vi "Begin.vi"(8 "error in (no error)":errorcluster, 10 "Settings":variant, 11 "Elevator Concrete in":refnum<class "Elevator Arm.lvclass">) -> (0 "error out":errorcluster, 3 "Elevator Concrete out":refnum<class "Elevator Arm.lvclass">)   [LabVIEW 2018, in "Elevator.lvlib" / "Elevator Arm.lvclass"]
doc: "Opens references and configures Elevator Arm resources."
uses:
  Elevator Arm.lvclass
  C:/Users/Public/Documents/2019DeepSpace/Classes/Elevator/Elevator.lvclass
  <vilib>/Rock Robotics/WPI/ThirdParty/Phoenix-LabVIEW/Motor Controller/Controls/CTRE_Phoenix_MotorControl_EnhancedMotorControllerConfigurables.ctl
  <vilib>/Rock Robotics/WPI/ThirdParty/Phoenix-LabVIEW/Motor Controller/Controls/CTRE_Phoenix_MotorControl_BaseConfigurables.ctl
  <vilib>/Rock Robotics/WPI/ThirdParty/Phoenix-LabVIEW/Motor Controller/Controls/CTRE_Phoenix_MotorControl_VelocityMeasurementPeriod.ctl
  <vilib>/Rock Robotics/WPI/ThirdParty/Phoenix-LabVIEW/Motor Controller/Controls/CTRE_Phoenix_MotorControl_SlotStructure.ctl
  <vilib>/Rock Robotics/WPI/ThirdParty/Phoenix-LabVIEW/Motor Controller/Controls/CTRE_Phoenix_MotorControl_FilterStruct.ctl
  <vilib>/Rock Robotics/WPI/ThirdParty/Phoenix-LabVIEW/Motor Controller/Controls/CTRE_Phoenix_MotorControl_RemoteSourceType.ctl
  <vilib>/Rock Robotics/WPI/ThirdParty/Phoenix-LabVIEW/Controls/CTRE_Phoenix_CustomParamConfiguration.ctl
  <vilib>/Rock Robotics/WPI/ThirdParty/Phoenix-LabVIEW/Motor Controller/Controls/CTRE_Phoenix_MotorControl_FeedbackDevice.ctl
  <vilib>/Rock Robotics/WPI/ThirdParty/Phoenix-LabVIEW/Motor Controller/Controls/CTRE_Phoenix_MotorControl_SensorTermFeedbackDevice_Enhanced.ctl
  <vilib>/Rock Robotics/WPI/ThirdParty/Phoenix-LabVIEW/Motor Controller/Controls/CTRE_Phoenix_MotorControl_LimitSwitchNormal.ctl
  <vilib>/Rock Robotics/WPI/ThirdParty/Phoenix-LabVIEW/Motor Controller/Controls/CTRE_Phoenix_MotorControl_LimitSwitchSource_Local.ctl
  Controls/Elevator Position.ctl
  Elevator Arm.lvclass/Elevator Arm.ctl
  Elevator.lvclass/Elevator.ctl
  Public Methods/Write Array.vi
  <vilib>/Rock Robotics/WPI/ThirdParty/Phoenix-LabVIEW/Motor Controller/Get/CTRE_Phoenix_MotorController_GetPulseWidthAll.vi
  Elevator.lvclass
panel:
  out "Pulse Width Rise-to-Rise Time (us)":i32
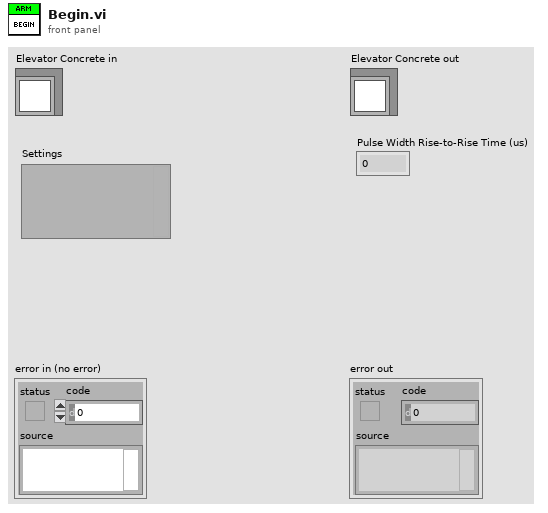
[diagram p1: front panel]
types:
  T1 = typedef "Elevator.lvlib/Elevator.lvclass/Elevator Position.ctl" = enum16{"CS, Cargo Ship Cargo", "C0, Cargo Ground", "C1, LV1 Cargo", "C2, LV2 Cargo", "C3, LV3 Cargo", "H0, LV1 Hatch", "H1, LV2 Hatch", "H2, LV3 Hatch"}
  T2 = typedef "CTRE_Phoenix_MotorControl_EnhancedMotorControllerConfigurables.ctl" = cluster{"Base Configurables":T3, "primaryPID":cluster{"selectedFeedbackCoefficient":dbl, "selectedFeedbackSensor":T9}, "auxiliaryPID":cluster{"selectedFeedbackCoefficient":dbl, "selectedFeedbackSensor":T9}, "sum0Term":T10, "sum1Term":T10, "diff0Term":T10, "diff1Term":T10, "forwardLimitSwitchNormal":T11, "reverseLimitSwitchNormal":T11, "forwardLimitSwitchDeviceID":i32, "reverseLimitSwitchDeviceID":i32, "forwardLimitSwitchSource":T12, "reverseLimitSwitchSource":T12, "peakCurrentLimit":i32, "peakCurrentDuration":i32, "continuousCurrentLimit":i32}
  T3 = typedef "CTRE_Phoenix_MotorControl_BaseConfigurables.ctl" = cluster{"openLoopRamp":dbl, "closedLoopRamp":dbl, "peakOutputForward":dbl, "peakOutputReverse":dbl, "nominalOutputForward":dbl, "nominalOutputReverse":dbl, "neutralDeadband":dbl, "voltageCompSaturation":dbl, "voltageMeasurementFilter":i32, "velocityMeasurementPeriod":T4, "velocityMeasurementWindow":i32, "forwardSoftLimitThreshold":i32, "reverseSoftLimitThreshold":i32, "forwardSoftLimitEnable":bool, "reverseSoftLimitEnable":bool, "slot0":T5, "slot1":T5, "slot2":T5, "slot3":T5, "auxPIDPolarity":bool, "remoteFilter0":T6, "remoteFilter1":T6, "motionCruiseVelocity":i32, "motionAcceleration":i32, "motionProfileTrajectoryPeriod":i32, "feedbackNotContinuous":bool, "remoteSensorClosedLoopDisableNeutralOnLOS":bool, "clearPositionOnLimitF":bool, "clearPositionOnLimitR":bool, "clearPositionOnQuadIdx":bool, "limitSwitchDisableNeutralOnLOS":bool, "softLimitDisableNeutralOnLOS":bool, "pulseWidthPeriod_EdgesPerRot":i32, "pulseWidthPeriod_FilterWindowSz":i32, "customParam":T8, "trajectoryInterpolationEnable":bool}
  T4 = typedef "CTRE_Phoenix_MotorControl_VelocityMeasurementPeriod.ctl" = u16
  T5 = typedef "CTRE_Phoenix_MotorControl_SlotStructure.ctl" = cluster{"P":dbl, "I":dbl, "D":dbl, "F":dbl, "integralZone":dbl, "allowableClosedLoopError":i32, "maxIntegralAccumulator":dbl, "closedLoopPeakOutput":dbl, "closedLoopPeriod":i32}
  T6 = typedef "CTRE_Phoenix_MotorControl_FilterStruct.ctl" = cluster{"remoteSensorDeviceID":u8, "remoteSensorSource":T7}
  T7 = typedef "CTRE_Phoenix_MotorControl_RemoteSourceType.ctl" = enum16{"Off", "Talon SRX Selected Sensor", "Pigeon IMU Yaw", "Pigeon IMU Pitch", "Pigeon IMU Roll", "CANifier Quadrature", "CANifier PWM Input 0", "CANifier PWM Input 1", "CANifier PWM Input 2", "CANifier PWM Input 3", "Gadgeteer Pigeon Yaw", "Gadgeteer Pigeon Pitch", "Gadgeteer Pigeon Roll"}
  T8 = typedef "CTRE_Phoenix_CustomParamConfiguration.ctl" = cluster{"customParam0":i32, "customParam1":i32}
  T9 = typedef "CTRE_Phoenix_MotorControl_FeedbackDevice.ctl" = i8
  T10 = typedef "CTRE_Phoenix_MotorControl_SensorTermFeedbackDevice_Enhanced.ctl" = i8
  T11 = typedef "CTRE_Phoenix_MotorControl_LimitSwitchNormal.ctl" = enum16{"Normally Open", "Normally Closed", "Disabled"}
  T12 = typedef "CTRE_Phoenix_MotorControl_LimitSwitchSource_Local.ctl" = enum16{"Feedback Connector", "Remote Talon SRX", "Remote CANifier", "Deactivated"}
  T13 = typedef "Elevator.lvlib/Elevator.lvclass/Elevator IDs.ctl" = cluster{"Wrist":u8, "Left Master":u8, "Left Slave":u8, "Right Master":u8, "Right Slave":u8, "Vacumm Pump 1":u8, "Vacumm Pump 2":u8, "Elevator Linear Master":u8, "Elevator Linear Slave":u8}
  T14 = typedef "Elevator.lvlib/Elevator.lvclass/Elevator Constants.ctl" = cluster{"Arm Motion Magic Max Velocity":u32, "Arm Motion Magic Max Acceleration":u32, "Wrist Motion Magic Max Velocity":u32, "Wrist Motion Magic Max Acceleration":u32, "Elevator Linear Motion Magic Max Velocity":u32, "Elevator Linear Motion Magic Max Acceleration":u32, "Arm Gear Ratio":dbl, "Wrist Gear Ratio":dbl, "Elevator Linear Gear Ratio":dbl, "Arm Encoder ABS Value":i32, "Wrist Encoder ABS Value":i32}
  T15 = typedef "WPI_MotorControlDeviceRef.ctl" = cluster{"DeviceStatus":errorcluster, "Type":T16, "PWM":cluster{"PWM Channel":T17, "DeadBand":T18}, "CAN":cluster{"Device Number":u8, "SetOutput VI Ref":variant, "GetOutput VI Ref":variant, "Enable VI Ref":variant, "Disable VI Ref":variant, "Data":variant}, "Invert":bool, "DIO PWM":cluster{"PWM \"Enable\" Channel":T17, "DIOChannel":T19, "PWM Rate":dbl}}
  T16 = typedef "WPI_MotorControlType.ctl" = enum16{"PWM", "CAN", "DIO PWM"}
  T17 = typedef "FPGA_DIOPWMChannel.ctl" = enum8{"PWM 0", "PWM 1", "PWM 2", "PWM 3", "PWM 4", "PWM 5", "PWM 6", "PWM 7", "PWM 8", "PWM 9", "PWM MXP 0", "PWM MXP 1", "PWM MXP 2", "PWM MXP 3", "PWM MXP 4", "PWM MXP 5", "PWM MXP 6", "PWM MXP 7", "PWM MXP 8", "PWM MXP 9", "Invalid"}
  T18 = typedef "WPI_PWMDeadband.ctl" = cluster{"Name":string, "maxPositivePwm":i32, "minPositivePwm":i32, "centerPwm":i32, "maxNegativePwm":i32, "minNegativePwm":i32, "angularRange":u16}
  T19 = typedef "FPGA_DIOChannel.ctl" = enum8{"DIO 0", "DIO 1", "DIO 2", "DIO 3", "DIO 4", "DIO 5", "DIO 6", "DIO 7", "DIO 8", "DIO 9", "DIO MXP 0", "DIO MXP 1", "DIO MXP 2", "DIO MXP 3", "DIO MXP 4", "DIO MXP 5", "DIO MXP 6", "DIO MXP 7", "DIO MXP 8", "DIO MXP 9", "DIO MXP 10", "DIO MXP 11", "DIO MXP 12", "DIO MXP 13", "DIO MXP 14", "DIO MXP 15", "SPI Port CS1", "SPI Port CS2", "SPI Port CS3", "SPI Port MISO", "SPI Port MOSI", "Invalid"}
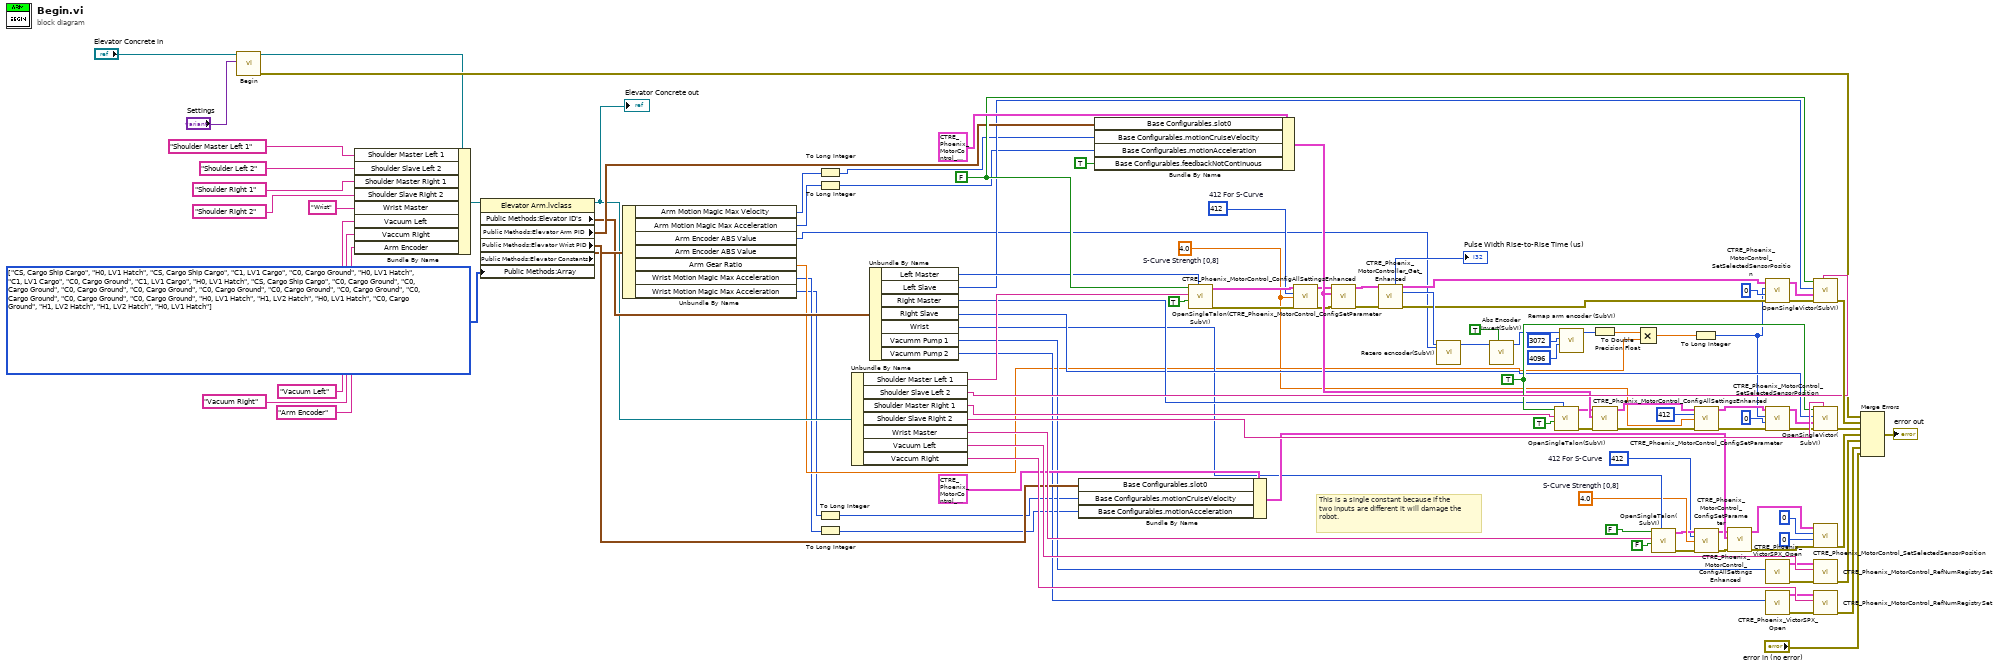
[diagram p0: block diagram]
diagram:
  w12 = T1[][] [[enum."CS, Cargo Ship Cargo", enum."H0, LV1 Hatch", enum."CS, Cargo Ship Cargo", enum."C1, LV1 Cargo"], [enum."C0, Cargo Ground", enum."H0, LV1 Hatch", enum."C1, LV1 Cargo", enum."C0, Cargo Ground"], [enum."C1, LV1 Cargo", enum."H0, LV1 Hatch", enum."CS, Cargo Ship Cargo", enum."C0, Cargo Ground"], [enum."C0, Cargo Ground", enum."C0, Cargo Ground", enum."C0, Cargo Ground", enum."C0, Cargo Ground"], [enum."C0, Cargo Ground", enum."C0, Cargo Ground", enum."C0, Cargo Ground", enum."C0, Cargo Ground"], [enum."C0, Cargo Ground", enum."H0, LV1 Hatch", enum."H1, LV2 Hatch", enum."H0, LV1 Hatch"], [enum."C0, Cargo Ground", enum."H1, LV2 Hatch", enum."H1, LV2 Hatch", enum."H0, LV1 Hatch"]] items=["CS, Cargo Ship Cargo", "C0, Cargo Ground", "C1, LV1 Cargo", "C2, LV2 Cargo", "C3, LV3 Cargo", "H0, LV1 Hatch", "H1, LV2 Hatch", "H2, LV3 Hatch"] ("Array")
  w22 = u16 412  # 412 For S-Curve
  w23 = u32 412  # 412 For S-Curve
  w31 = 4.0  # S-Curve Strength [0,8]
  w1 = 4.0  # S-Curve Strength [0,8]
  w72 = FALSE ("invert")
  w88 = TRUE ("Invert?")
  # "This is a single constant because if the two inputs are different it will damage the robot."
  n1 = call-parent "Begin.vi"("Settings"="Settings", "Elevator in"="Elevator Concrete in") -> ("error out"=w16:errorcluster, "Elevator out"=w14:refnum<class "Elevator Arm.lvclass">)  [unwired: 8 in]
  n2 = Bundle By Name(cluster=w14, "Shoulder Master Left 1"="Shoulder Master Left 1" ("Shoulder Slave Left 1"), "Shoulder Slave Left 2"="Shoulder Left 2", "Shoulder Master Right 1"="Shoulder Right 1", "Shoulder Slave Right 2"="Shoulder Right 2", "Wrist Master"="Wrist", "Vacuum Left"="Vacuum Left", "Vaccum Right"="Vacuum Right", "Arm Encoder"="Arm Encoder") -> (w67:refnum<class "Elevator Arm.lvclass">)
  n3 = property class="Elevator Arm.lvclass"(reference=w67, "Public Methods:Array"=w12) -> (reference out=w13:refnum<class "Elevator Arm.lvclass">, "Public Methods:Elevator ID's"=w61:T13, "Public Methods:Elevator Arm PID"=w66:T5, "Public Methods:Elevator Wrist PID"=w65:T5, "Public Methods:Elevator Constants"=w64:T14)  [unwired: 1 in, 1 out]
  "Elevator Concrete out" <- w13
  n4 = Unbundle By Name(w64) -> ("Arm Motion Magic Max Velocity"=w63:u32, "Arm Motion Magic Max Acceleration"=w62:u32, "Arm Encoder ABS Value"=w4:i32, "Arm Gear Ratio"=w5:dbl, "Wrist Motion Magic Max Acceleration"=w3:u32, "Wrist Motion Magic Max Acceleration"=w2:u32)  [unwired: 1 out]
  n5 = To Long Integer(number=w63) -> (32bit integer=w9:i32)
  n6 = To Long Integer(number=w62) -> (32bit integer=w8:i32)
  n7 = To Long Integer(number=w2) -> (32bit integer=w6:i32)
  n8 = To Long Integer(number=w3) -> (32bit integer=w7:i32)
  n9 = Unbundle By Name(w13) -> ("Shoulder Master Left 1"=w106:string, "Shoulder Slave Left 2"=w105:string, "Shoulder Master Right 1"=w104:string, "Shoulder Slave Right 2"=w103:string, "Wrist Master"=w102:string, "Vacuum Left"=w101:string, "Vaccum Right"=w100:string)
  n10 = Unbundle By Name(w61) -> ("Left Master"=w58:u8, "Left Slave"=w57:u8, "Right Master"=w56:u8, "Right Slave"=w55:u8, "Wrist"=w54:u8, "Vacumm Pump 1"=w59:u8, "Vacumm Pump 2"=w60:u8)
  n11 = Bundle By Name(cluster=T2 {"Base Configurables"={"openLoopRamp"=0.0, "closedLoopRamp"=0.0, "peakOutputForward"=1.0, "peakOutputReverse"=-1.0, "nominalOutputForward"=0.0, "nominalOutputReverse"=0.0, "neutralDeadband"=0.04, "voltageCompSaturation"=0.0, "voltageMeasurementFilter"=32, "velocityMeasurementPeriod"=100, "velocityMeasurementWindow"=64, "forwardSoftLimitThreshold"=0, "reverseSoftLimitThreshold"=0, "forwardSoftLimitEnable"=FALSE, "reverseSoftLimitEnable"=FALSE, "slot0"={"P"=0.0, "I"=0.0, "D"=0.0, "F"=0.0, "integralZone"=0.0, "allowableClosedLoopError"=0, "maxIntegralAccumulator"=0.0, "closedLoopPeakOutput"=1.0, "closedLoopPeriod"=1}, "slot1"={"P"=0.0, "I"=0.0, "D"=0.0, "F"=0.0, "integralZone"=0.0, "allowableClosedLoopError"=0, "maxIntegralAccumulator"=0.0, "closedLoopPeakOutput"=1.0, "closedLoopPeriod"=1}, "slot2"={"P"=0.0, "I"=0.0, "D"=0.0, "F"=0.0, "integralZone"=0.0, "allowableClosedLoopError"=0, "maxIntegralAccumulator"=0.0, "closedLoopPeakOutput"=1.0, "closedLoopPeriod"=1}, "slot3"={"P"=0.0, "I"=0.0, "D"=0.0, "F"=0.0, "integralZone"=0.0, "allowableClosedLoopError"=0, "maxIntegralAccumulator"=0.0, "closedLoopPeakOutput"=1.0, "closedLoopPeriod"=1}, "auxPIDPolarity"=FALSE, "remoteFilter0"={"remoteSensorDeviceID"=0, "remoteSensorSource"=enum."Off"}, "remoteFilter1"={"remoteSensorDeviceID"=0, "remoteSensorSource"=enum."Off"}, "motionCruiseVelocity"=0, "motionAcceleration"=0, "motionProfileTrajectoryPeriod"=0, "feedbackNotContinuous"=FALSE, "remoteSensorClosedLoopDisableNeutralOnLOS"=FALSE, "clearPositionOnLimitF"=FALSE, "clearPositionOnLimitR"=FALSE, "clearPositionOnQuadIdx"=FALSE, "limitSwitchDisableNeutralOnLOS"=FALSE, "softLimitDisableNeutralOnLOS"=FALSE, "pulseWidthPeriod_EdgesPerRot"=1, "pulseWidthPeriod_FilterWindowSz"=1, "customParam"={"customParam0"=0, "customParam1"=0}, "trajectoryInterpolationEnable"=TRUE}, "primaryPID"={"selectedFeedbackCoefficient"=1.0, "selectedFeedbackSensor"=0}, "auxiliaryPID"={"selectedFeedbackCoefficient"=1.0, "selectedFeedbackSensor"=0}, "sum0Term"=0, "sum1Term"=0, "diff0Term"=0, "diff1Term"=0, "forwardLimitSwitchNormal"=enum."Normally Open", "reverseLimitSwitchNormal"=enum."Normally Open", "forwardLimitSwitchDeviceID"=0, "reverseLimitSwitchDeviceID"=0, "forwardLimitSwitchSource"=enum."Feedback Connector", "reverseLimitSwitchSource"=enum."Feedback Connector", "peakCurrentLimit"=1, "peakCurrentDuration"=1, "continuousCurrentLimit"=1} ("Enhanced Motor Controller Configurables"), "Base Configurables.slot0"=w65, "Base Configurables.motionCruiseVelocity"=w6, "Base Configurables.motionAcceleration"=w7) -> (w75:T2)
  n12 = Bundle By Name(cluster=T2 {"Base Configurables"={"openLoopRamp"=0.0, "closedLoopRamp"=0.0, "peakOutputForward"=1.0, "peakOutputReverse"=-1.0, "nominalOutputForward"=0.0, "nominalOutputReverse"=0.0, "neutralDeadband"=0.04, "voltageCompSaturation"=0.0, "voltageMeasurementFilter"=32, "velocityMeasurementPeriod"=100, "velocityMeasurementWindow"=64, "forwardSoftLimitThreshold"=0, "reverseSoftLimitThreshold"=0, "forwardSoftLimitEnable"=FALSE, "reverseSoftLimitEnable"=FALSE, "slot0"={"P"=0.0, "I"=0.0, "D"=0.0, "F"=0.0, "integralZone"=0.0, "allowableClosedLoopError"=0, "maxIntegralAccumulator"=0.0, "closedLoopPeakOutput"=1.0, "closedLoopPeriod"=1}, "slot1"={"P"=0.0, "I"=0.0, "D"=0.0, "F"=0.0, "integralZone"=0.0, "allowableClosedLoopError"=0, "maxIntegralAccumulator"=0.0, "closedLoopPeakOutput"=1.0, "closedLoopPeriod"=1}, "slot2"={"P"=0.0, "I"=0.0, "D"=0.0, "F"=0.0, "integralZone"=0.0, "allowableClosedLoopError"=0, "maxIntegralAccumulator"=0.0, "closedLoopPeakOutput"=1.0, "closedLoopPeriod"=1}, "slot3"={"P"=0.0, "I"=0.0, "D"=0.0, "F"=0.0, "integralZone"=0.0, "allowableClosedLoopError"=0, "maxIntegralAccumulator"=0.0, "closedLoopPeakOutput"=1.0, "closedLoopPeriod"=1}, "auxPIDPolarity"=FALSE, "remoteFilter0"={"remoteSensorDeviceID"=0, "remoteSensorSource"=enum."Off"}, "remoteFilter1"={"remoteSensorDeviceID"=0, "remoteSensorSource"=enum."Off"}, "motionCruiseVelocity"=0, "motionAcceleration"=0, "motionProfileTrajectoryPeriod"=0, "feedbackNotContinuous"=FALSE, "remoteSensorClosedLoopDisableNeutralOnLOS"=FALSE, "clearPositionOnLimitF"=FALSE, "clearPositionOnLimitR"=FALSE, "clearPositionOnQuadIdx"=FALSE, "limitSwitchDisableNeutralOnLOS"=FALSE, "softLimitDisableNeutralOnLOS"=FALSE, "pulseWidthPeriod_EdgesPerRot"=1, "pulseWidthPeriod_FilterWindowSz"=1, "customParam"={"customParam0"=0, "customParam1"=0}, "trajectoryInterpolationEnable"=TRUE}, "primaryPID"={"selectedFeedbackCoefficient"=1.0, "selectedFeedbackSensor"=0}, "auxiliaryPID"={"selectedFeedbackCoefficient"=1.0, "selectedFeedbackSensor"=0}, "sum0Term"=0, "sum1Term"=0, "diff0Term"=0, "diff1Term"=0, "forwardLimitSwitchNormal"=enum."Normally Open", "reverseLimitSwitchNormal"=enum."Normally Open", "forwardLimitSwitchDeviceID"=0, "reverseLimitSwitchDeviceID"=0, "forwardLimitSwitchSource"=enum."Feedback Connector", "reverseLimitSwitchSource"=enum."Feedback Connector", "peakCurrentLimit"=1, "peakCurrentDuration"=1, "continuousCurrentLimit"=1} ("Enhanced Motor Controller Configurables"), "Base Configurables.slot0"=w66, "Base Configurables.motionCruiseVelocity"=w9, "Base Configurables.motionAcceleration"=w8, "Base Configurables.feedbackNotContinuous"=TRUE) -> (w86:T2)
  n13 = call "OpenSingleTalon(SubVI).vi"("can_id"=w58, "sensor_phase"=TRUE, "refnum name"=w106, "invert"=w72) -> ("error out"=w37:errorcluster, "PhoenixMotorControlDevRef"=w39:T15)  [unwired: 6 in]
  n14 = call <vilib>:"CTRE_Phoenix_MotorControl_ConfigSetParameter.vi"("PhoenixMotorControlDevRef"=w39, "Parameter"=w22, "value"=w1, "error in (no error)"=w37) -> ("PhoenixMotorControlDevRef"=w38:T15, "error out"=w36:errorcluster)  [unwired: 10 in]
  n15 = call <vilib>:"CTRE_Phoenix_MotorControl_ConfigAllSettingsEnhanced.vi"("error in (no error)"=w36, "Enhanced Motor Controller Configurables"=w86, "PhoenixMotorControlDevRef"=w38) -> ("error out"=w41:errorcluster, "PhoenixMotorControlDevRef"=w43:T15)  [unwired: 7 in]
  n16 = call-poly <vilib>:"CTRE_Phoenix_MotorController_Get_Enhanced.vi"("PhoenixMotorControlDevRef"=w43, "error in"=w41) -> ("Pulse Width Rise-to-Rise Time (us)"=→"Pulse Width Rise-to-Rise Time (us)":i32, "PhoenixMotorControlDevRef"=w42:T15, "Pulse Width Position"=w53:i32, "error out"=w40:errorcluster)  [unwired: 8 in, 2 out]
  n17 = call "Rezero ecncoder(SubVI).vi"("Zero"=w4, "Encoder"=w53) -> ("Rezeroed Encoder"=w44:i32)  [unwired: 9 in]
  n18 = call "Abs Encoder Invert(SubVI).vi"("Sensor Phase"=TRUE, "encoder"=w44) -> ("encoder reversed"=w46:i32)  [unwired: 9 in]
  n19 = call "OpenSingleTalon(SubVI).vi"("can_id"=w56, "sensor_phase"=TRUE, "refnum name"=w104, "invert"=w88) -> ("error out"=w89:errorcluster, "PhoenixMotorControlDevRef"=w68:T15)  [unwired: 6 in]
  n20 = call "Remap arm encoder (SubVI).vi"("encoder ticks per revolution"=4096, "crossover to negative"=3072, "Value"=w46) -> ("Mapped"=w49:i32)  [unwired: 8 in]
  n21 = To Double Precision Float(number=w49) -> (double precision float=w11:dbl)
  n22 = call <vilib>:"CTRE_Phoenix_MotorControl_ConfigAllSettingsEnhanced.vi"("error in (no error)"=w89, "Enhanced Motor Controller Configurables"=w86, "PhoenixMotorControlDevRef"=w68) -> ("error out"=w33:errorcluster, "PhoenixMotorControlDevRef"=w35:T15)  [unwired: 7 in]
  n23 = Multiply(x=w11, y=w5) -> (x*y=w50:dbl)
  n24 = call "OpenSingleTalon(SubVI).vi"("can_id"=w54, "sensor_phase"=FALSE, "refnum name"=w102, "invert"=FALSE) -> ("error out"=w28:errorcluster, "PhoenixMotorControlDevRef"=w30:T15)  [unwired: 6 in]
  n25 = To Long Integer(number=w50) -> (32bit integer=w10:i32)
  n26 = call <vilib>:"CTRE_Phoenix_MotorControl_ConfigSetParameter.vi"("PhoenixMotorControlDevRef"=w35, "Parameter"=u32 412 ("subValue"), "value"=w1, "error in (no error)"=w33) -> ("PhoenixMotorControlDevRef"=w34:T15, "error out"=w32:errorcluster)  [unwired: 10 in]
  n27 = call <vilib>:"CTRE_Phoenix_MotorControl_ConfigSetParameter.vi"("PhoenixMotorControlDevRef"=w30, "Parameter"=w23, "value"=w31, "error in (no error)"=w28) -> ("PhoenixMotorControlDevRef"=w29:T15, "error out"=w27:errorcluster)  [unwired: 10 in]
  n28 = call <vilib>:"CTRE_Phoenix_MotorControl_ConfigAllSettingsEnhanced.vi"("error in (no error)"=w27, "Enhanced Motor Controller Configurables"=w75, "PhoenixMotorControlDevRef"=w29) -> ("error out"=w76:errorcluster, "PhoenixMotorControlDevRef"=w25:T15)  [unwired: 7 in]
  n29 = call <vilib>:"CTRE_Phoenix_MotorControl_SetSelectedSensorPosition.vi"("error in (no error)"=w40, "pidLoopIdx"=u32 0, "New Sensor Position"=w10, "PhoenixMotorControlDevRef"=w42) -> ("error out"=w108:errorcluster, "PhoenixMotorControlDevRef"=w107:T15)  [unwired: 6 in]
  n30 = call <vilib>:"CTRE_Phoenix_MotorControl_SetSelectedSensorPosition.vi"("error in (no error)"=w32, "pidLoopIdx"=u32 0, "New Sensor Position"=w10, "PhoenixMotorControlDevRef"=w34) -> ("error out"=w91:errorcluster, "PhoenixMotorControlDevRef"=w90:T15)  [unwired: 6 in]
  n31 = call <vilib>:"CTRE_Phoenix_VictorSPX_Open.vi"("Device Number"=w59) -> ("error out"=w80:errorcluster, "CAN Talon SRX Ref"=w79:T15)  [unwired: 9 in]
  n32 = call <vilib>:"CTRE_Phoenix_VictorSPX_Open.vi"("Device Number"=w60) -> ("error out"=w83:errorcluster, "CAN Talon SRX Ref"=w82:T15)  [unwired: 9 in]
  n33 = call "OpenSingleVictor(SubVI).vi"("refnum name"=w105, "error in (no error)"=w108, "Master Controller to Follow"=w107, "Device Number"=w57, "Invert?"=w72) -> ("error out"=w109:errorcluster)  [unwired: 5 in, 1 out]
  n34 = call "OpenSingleVictor(SubVI).vi"("refnum name"=w103, "error in (no error)"=w91, "Master Controller to Follow"=w90, "Device Number"=w55, "Invert?"=w88) -> ("error out"=w92:errorcluster)  [unwired: 5 in, 1 out]
  n35 = call <vilib>:"CTRE_Phoenix_MotorControl_SetSelectedSensorPosition.vi"("error in (no error)"=w76, "pidLoopIdx"=u32 0 ("New Sensor Position"), "New Sensor Position"=0, "PhoenixMotorControlDevRef"=w25) -> ("error out"=w73:errorcluster)  [unwired: 6 in, 1 out]
  n36 = call <vilib>:"CTRE_Phoenix_MotorControl_RefNumRegistrySet.vi"("error in (no error)"=w80, "refnum name"=w101, "PhoenixMotorControlDevRef"=w79) -> ("error out"=w81:errorcluster)  [unwired: 7 in, 1 out]
  n37 = call <vilib>:"CTRE_Phoenix_MotorControl_RefNumRegistrySet.vi"("error in (no error)"=w83, "refnum name"=w100, "PhoenixMotorControlDevRef"=w82) -> ("error out"=w84:errorcluster)  [unwired: 7 in, 1 out]
  n38 = Merge Errors(w16, w109, w92, w73, w81, w84, "error in (no error)") -> (→"error out":errorcluster)
